vi "Storage Immediate Wrapper.vi"() -> ()   [LabVIEW 2019]
panel:
  in  "Synchronication":enum16{"Start", "Wait"}(ring)
  in  "Setpoint":dbl
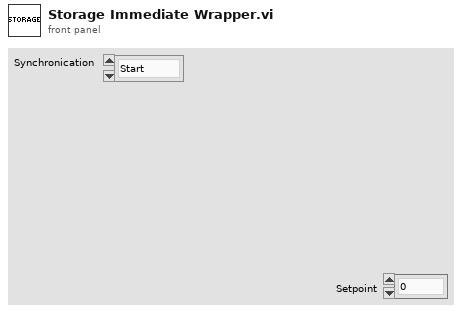
[diagram p1: front panel]
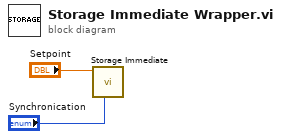
[diagram p0: block diagram]
diagram:
  n1 = call "Storage Immediate.vi"("Synchronication"="Synchronication", "Setpoint"="Setpoint") -> ()  [unwired: 9 in, 1 out]
